vi "globalEventos.vi"() -> ()   [LabVIEW 2018]
panel:
  out "Eventos":string
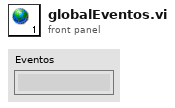
[diagram p1: front panel]
diagram:
